vi "INI Session.vi"(11 "Section Name(\"\" as Default)":string) -> (3 "App.Name":string)   [LabVIEW 2017, in "INI-Static-Variable-Support.lvlib"]
uses:
  INI-Static-Variable-Support.lvlib
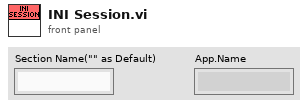
[diagram p1: front panel]
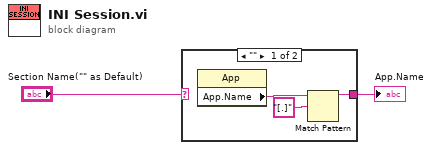
[diagram p0: block diagram]
diagram:
  n1 = case shown="\"\"" "Section Name(\"\" as Default)" {
    selector: "Section Name(\"\" as Default)" -> [_ w6]
    tunnel: [w3 w6] -> w2
    frame "" {
      n2 = property class="App"() -> ("App.Name"=w4:string)  [unwired: 2 in, 2 out]
      n3 = Match Pattern(string=w4, regular expression="[.]") -> (before substring=w3:string)  [unwired: 1 in, 3 out]
    }
    frame Default {
    }
  }
  "App.Name" <- w2
